vi "Get Parent Banner Icon.vi"(8 "error in (no error)":errorcluster, 11 "QControl Creation in":refnum<class "QControl Creation.lvclass">) -> (0 "error out":errorcluster, 2 "Banner BG Color":u32(colorbox), 3 "Banner Text Color":u32(colorbox))   [LabVIEW 2015, in "QControl Creation.lvclass"]
doc: "<b> </b> <b> </b>\n©2016 Q Software Innovations, LLC (QSI)\nwritten by Quentin Alldredge\nproduced in LabVIEW 2015\n\nsupport@qsoftwareinnovations.com\nwww.qsoftwareinnovations.com\n\nAll rights reserved.\n\nRedistribution and use in source and binary forms, with or without modification, are permitted provided that the following conditions are met:\n\n * Redistributions of source code must retain the above copyright notice, this list of conditions and the following disclaimer.\n * Redistributions in binary form must reproduce the above copyright notice, this list of conditions and the following disclaimer in the documentation and/or other materials provided with the distribution.\n * Neither the name of Q Software Innovations, LLC. nor the names of its contributors may be used to endorse or promote products derived from this software without specific prior written permission.\n\nTHIS SOFTWARE IS PROVIDED BY THE COPYRIGHT HOLDERS AND CONTRIBUTORS \"AS IS\" AND ANY EXPRESS OR IMPLIED WARRANTIES, INCLUDING, BUT NOT LIMITED TO, THE IMPLIED WARRANTIES OF MERCHANTABILITY AND FITNESS FOR A PARTICULAR PURPOSE ARE DISCLAIMED. IN NO EVENT SHALL THE COPYRIGHT OWNER OR CONTRIBUTORS BE LIABLE FOR ANY DIRECT, INDIRECT, INCIDENTAL, SPECIAL, EXEMPLARY, OR CONSEQUENTIAL DAMAGES (INCLUDING, BUT NOT LIMITED TO, PROCUREMENT OF SUBSTITUTE GOODS OR SERVICES; LOSS OF USE, DATA, OR PROFITS; OR BUSINESS INTERRUPTION) HOWEVER CAUSED AND ON ANY THEORY OF LIABILITY, WHETHER IN CONTRACT, STRICT LIABILITY, OR TORT (INCLUDING NEGLIGENCE OR OTHERWISE) ARISING IN ANY WAY OUT OF THE USE OF THIS SOFTWARE, EVEN IF ADVISED OF THE POSSIBILITY OF SUCH DAMAGE."
uses:
  QControl Creation.lvclass
  <vilib>/LabVIEW Icon API/LabVIEW Icon API.lvlib
  <vilib>/LabVIEW Icon API/lv_icon/Classes/Icon/Icon.lvclass
  <vilib>/LabVIEW Icon API/lv_icon/Classes/Icon Framework/Icon Framework.lvclass
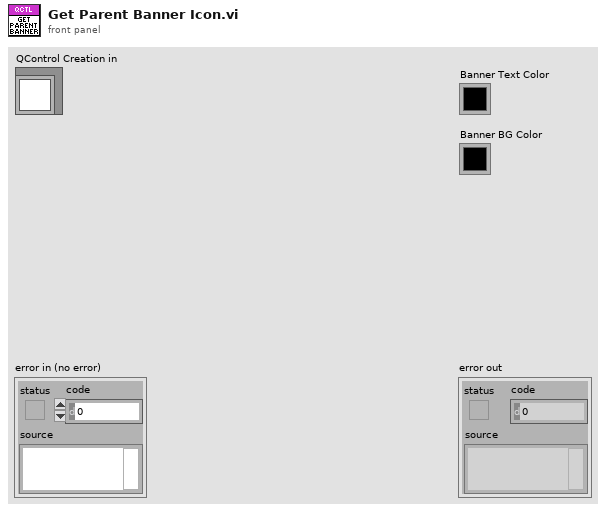
[diagram p1: front panel]
types:
  T1 = typedef "imagedata.ctl" = cluster{"image type":i32, "image depth":i32, "image":u8[], "mask":u8[], "colors":u32[], "Rectangle":cluster{"left":i16, "top":i16, "right":i16, "bottom":i16}}
  T2 = typedef "BodyText.ctl" = cluster{"Line 1 text":string, "Line 2 text":string, "Line 3 text":string, "Line 4 text":string, "Line 1 color":u32, "Line 2 color":u32, "Line 3 color":u32, "Line 4 color":u32, "Body Text Spec":cluster{"Font":T3, "Alignment":T4, "Size":u8}, "Center text vertically":bool, "Capitalize Text":bool}
  T3 = typedef "Font.ctl" = string
  T4 = typedef "Alignment.ctl" = u16
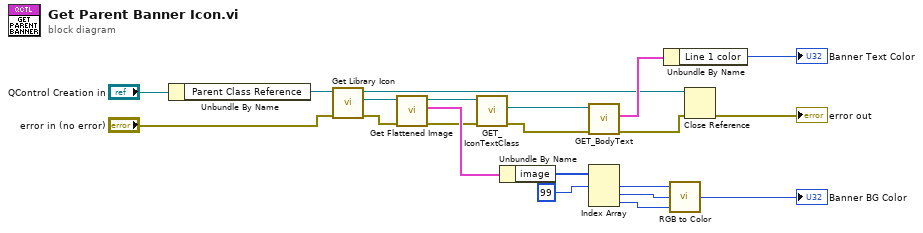
[diagram p0: block diagram]
diagram:
  n1 = Unbundle By Name("QControl Creation in") -> ("Parent Class Reference"=w1:refnum<vi>)
  n2 = call <vilib>:"Get Library Icon.vi"("error in (no error)"="error in (no error)", "Library Refnum in"=w1) -> ("error out"=w19:errorcluster, "Icon"=w7:refnum<class "Icon.lvclass">, "Library Refnum out"=w6:refnum<vi>)  [unwired: 7 in]
  n3 = call <vilib>:"Get Flattened Image.vi"("error in (no error)"=w19, "lv_icon.lvlib:Icon.lvclass in"=w7) -> ("error out"=w9:errorcluster, "Color Image"=w18:T1, "lv_icon.lvlib:Icon.lvclass out"=w17:refnum<class "Icon.lvclass">)  [unwired: 6 in, 1 out]
  n4 = call-dynamic "GET_IconTextClass.vi"("error in (no error)"=w9, "Icon.lvclass in"=w17) -> ("error out"=w8:errorcluster, "Icon Framework.lvclass"=w16:refnum<class "Icon Framework.lvclass">)  [unwired: 7 in, 1 out]
  n5 = Unbundle By Name(w18) -> ("image"=w14:u8[])
  n6 = call-dynamic "GET_BodyText.vi"("error in (no error)"=w8, "Icon Framework.lvclass in"=w16) -> ("error out"=w5:errorcluster, "Body Text"=w15:T2)  [unwired: 6 in, 2 out]
  n7 = Index Array(array=w14, index #1=99) -> (element #1=w12:u8, element #2=w11:u8, element #3=w10:u8)  [unwired: 2 in]
  n8 = Unbundle By Name(w15) -> ("Line 1 color"=→"Banner Text Color":u32)
  n9 = call <vilib>:"RGB to Color.vi"("B"=w10, "G"=w11, "R"=w12) -> ("Color"=→"Banner BG Color":u32)
  n10 = Close Reference(reference=w6, error in (no error)=w5) -> (error out=→"error out":errorcluster)
